vi "Endpoint Connected.vi"(8 "error in":errorcluster, 10 "Endpoint":refnum<class "Message Enqueuer.lvclass">, 11 "Study Actor in":refnum<class "Study Actor.lvclass">) -> (0 "error out":errorcluster, 3 "Study Actor out":refnum<class "Study Actor.lvclass">)   [LabVIEW 2023, in "HAL GOOP4.lvlib" / "Study Actor.lvlib" / "Study Actor.lvclass"]
doc: "Override this method to specify how the receiving actor responds to a Connected message from a nested endpoint actor."
uses:
  Study Actor.lvclass
  <vilib>/ActorFramework/Message Enqueuer/Message Enqueuer.lvclass
  Study Actor.lvclass/Study Actor.ctl
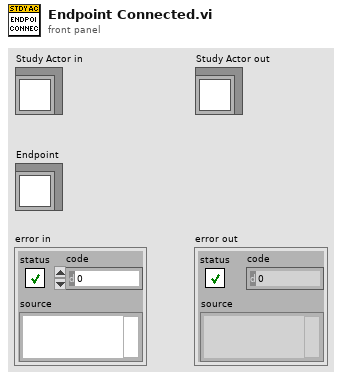
[diagram p1: front panel]
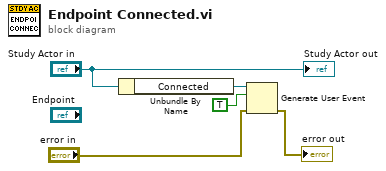
[diagram p0: block diagram]
diagram:
  n1 = Unbundle By Name("Study Actor in") -> ("Connected"=w4:refnum<user-event>)
  n2 = Generate User Event(user event=w4, event data cluster=TRUE, error in="error in") -> (error out=→"error out":errorcluster)  [unwired: 1 in, 1 out]
  "Study Actor out" <- "Study Actor in"
